vi "Close.vi"(8 "Error In":errorcluster, 11 "Sequencer In":refnum<class "Sequencer.lvclass">) -> (0 "Error Out":errorcluster)   [LabVIEW 2019, in "Sequencer.lvclass"]
uses:
  Sequencer.lvclass
  Process/Process.lvclass
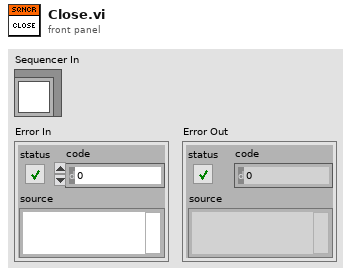
[diagram p1: front panel]
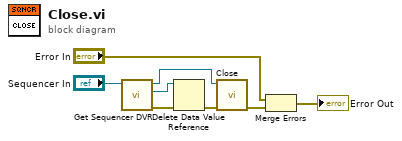
[diagram p0: block diagram]
diagram:
  n1 = call "Get Sequencer DVR.vi"("Sequencer In"="Sequencer In") -> ("Error Out"=w1:errorcluster, "DVR"=w4:refnum<data-value>, "Sequencer Out"=w3:refnum<class "Sequencer.lvclass">)  [unwired: 8 in]
  n2 = Delete Data Value Reference(data value reference=w4, error in=w1) -> (error out=w2:errorcluster)  [unwired: 1 out]
  n3 = call-parent "Close.vi"("Error In"=w2, "Process In"=w3) -> ("Error Out"=w8:errorcluster)  [unwired: 9 in]
  n4 = Merge Errors("Error In", w8) -> (→"Error Out":errorcluster)
